vi "Get Cluster Elements.vi"(8 "Error In":errorcluster, 10 "Cluster":variant, 11 "Type Enum (Cluster)":T1=enum."Cluster") -> (0 "Error Out":errorcluster, 2 "Cluster Elements":variant[](array[variant]))   [LabVIEW 2020]
doc: "This VI was created for use with the Read/Write Cluster VIs. It breaks a cluster up into its individual elements and passes the elements out in an array of variants.\n\nFreeware from Moore Good Ideas, www.mooregoodideas.com. Do not remove this line."
uses:
  <vilib>/Utility/VariantDataType/Type.ctl
  <vilib>/Utility/VariantDataType/VariantType.lvlib
panel:
  out "Numeric":i32
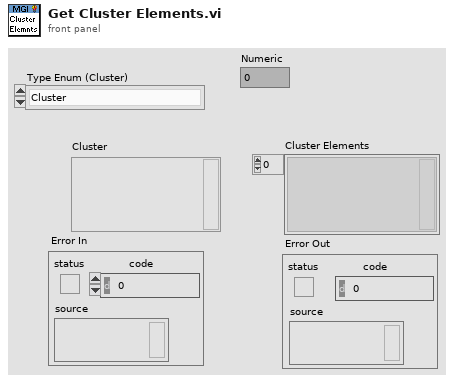
[diagram p1: front panel]
types:
  T1 = typedef "VariantType.lvlib/Type.ctl" = enum8{"Invalid Type", "Void", "I8", "I16", "I32", "I64", "U8", "U16", "U32", "U64", "Single Float", "Double Float", "Extended Float", "Single Complex", "Double Complex", "Extended Complex", "Enum U8", "Enum U16", "Enum U32", "Enum U64", "Single Float With Unit", "Double Float With Unit", "Extended Float With Unit", "Single Complex with Unit", "Double Complex with Unit", "Extended Complex with Unit", "Boolean", "String", "Path", "Picture", "Tag", "Array", "Cluster", "Variant", "LV Variant", "Waveform", "Timestamp", "Digital Waveform", "Digital Data", "ExpressData", "Refnum", "External Data", "VI", "Poly VI", "LabVIEW Class Instance", "Fixed Point"}
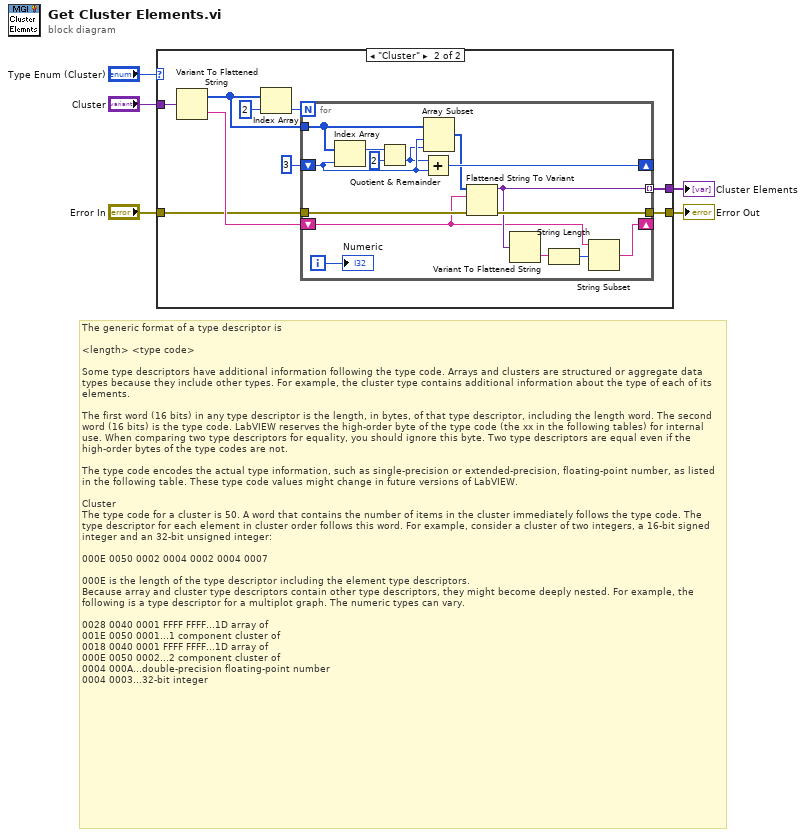
[diagram p0: block diagram]
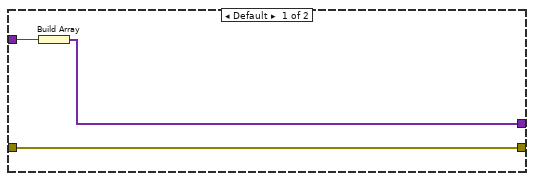
[diagram p2: hidden frame]
diagram:
  # "The generic format of a type descriptor is\n\n<length> <type code> \n\nSome type descriptors have additional information following the type code. Arrays and clusters are structured or aggregate data types because they include other types. For example, the cluster type contains additional information about the type of each of its elements.\n\nThe first word (16 bits) in any type descriptor is the length, in bytes, of that type descriptor, including the length word. The second word (16 bits) is the type code. LabVIEW reserves the high-order byte of the type code (the xx in the following tables) for internal use. When comparing two type descriptors for equality, you should ignore this byte. Two type descriptors are equal even if the high-order bytes of the type codes are not.\n\nThe type code encodes the actual type information, such as single-precision or extended-precision, floating-point number, as listed in the following table. These type code values might change in future versions of LabVIEW.\n\nCluster\nThe type code for a cluster is 50. A word that contains the number of items in the cluster immediately follows the type code. The type descriptor for each element in cluster order follows this word. For example, consider a cluster of two integers, a 16-bit signed integer and an 32-bit unsigned integer:\n\n000E 0050 0002 0004 0002 0004 0007 \n\n000E is the length of the type descriptor including the element type descriptors.\nBecause array and cluster type descriptors contain other type descriptors, they might become deeply nested. For example, the following is a type descriptor for a multiplot graph. The numeric types can vary.\n\n0028 0040 0001 FFFF FFFF...1D array of\n001E 0050 0001...1 component cluster of \n0018 0040 0001 FFFF FFFF...1D array of\n000E 0050 0002...2 component cluster of \n0004 000A...double-precision floating-point number \n0004 0003...32-bit integer"
  n1 = case shown="\"Cluster\"" "Type Enum (Cluster)" {
    tunnel: [w8 w10] -> w5
    tunnel: "Error In" -> [w8 w11]
    tunnel: "Cluster" -> [w7 w12]
    tunnel: [w6 w9] -> w1
    frame Default {
      n2 = Build Array(w7) -> (w6:variant[])
    }
    frame "Cluster" {
      n3 = Variant To Flattened String(Variant=w12) -> (data string=w17:string, 1:w14:i16[])
      n4 = Index Array(array=w14, index=2) -> (element=w16:i16)
      n5 = for {
        N: w16 -> [_]
        shift-right: [w31] -> _
        shift-left: 3 ("Index") -> [w30]
        tunnel: w14 -> [w32]
        tunnel: w11 -> [w25]
        tunnel: [w24] -> w10
        tunnel: [w22] -> w9 mode=indexing
        shift-right: [w20] -> _
        shift-left: w17 -> [w19]
        i -> [w18]
        n6 = Index Array(array=w32, index=w30) -> (element=w28:i16)
        n7 = Quotient & Remainder(x=w28, y=i16 2) -> (floor(x/y)=w29:i16)  [unwired: 1 out]
        n8 = Add(x=w29, y=w30) -> (x+y=w31:i32)
        n9 = Array Subset(array=w32, index=w30, length=w29) -> (w26:i16[])
        n10 = Flattened String To Variant(4:w25, 6:w19, 7:w26) -> (0:w24:errorcluster, 3:w22:variant)
        n11 = Variant To Flattened String(Variant=w22) -> (data string=w23:string)  [unwired: 1 out]
        n12 = String Length(string=w23) -> (length=w21:i32)
        n13 = String Subset(string=w19, offset (0)=w21) -> (substring=w20:string)  [unwired: 1 in]
        "Numeric" <- w18
      }
    }
  }
  "Error Out" <- w5
  "Cluster Elements" <- w1
